vi "Create Case Structure (Boolean).vi"(0 "Diagram in":refnum<vi>, 2 "location (0, 0)":T1, 5 "Selector":refnum<vi>, 7 "Inputs":refnum<vi>[](array[refnum]), 11 "error in (no error)":errorcluster) -> (4 "Selected Diagram":refnum<vi>, 6 "Selector":refnum<vi>, 8 "Inputs":refnum<vi>[](array[refnum]), 15 "error out":errorcluster)   [LabVIEW 2015, in "Scripting.lvlib"]
doc: "Creates a Case Structure at <B>location</B> on <B>Diagram in</B> with True and False cases, in that order."
uses:
  Scripting.lvlib
  <vilib>/Utility/miscctls.llb/LVPointTypeDef.ctl
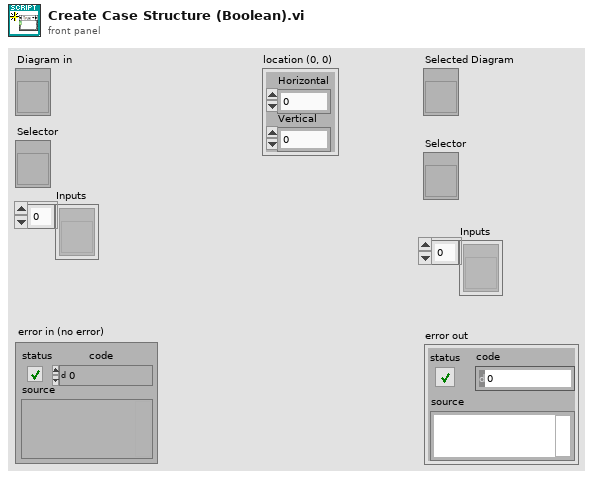
[diagram p1: front panel]
types:
  T1 = typedef "LVPointTypeDef.ctl" = cluster{"Horizontal":i16, "Vertical":i16}
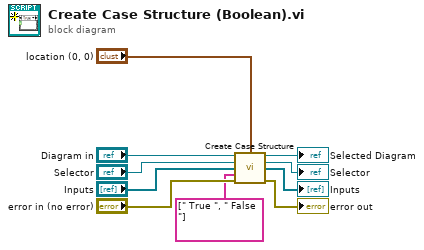
[diagram p0: block diagram]
diagram:
  n1 = call "Create Case Structure.vi"("Diagram in"="Diagram in", "location (0, 0)"="location (0, 0)", "Selector"="Selector", "Inputs"="Inputs", "Frames"=string[] [" True ", " False "], "error in (no error)"="error in (no error)") -> ("Selected Diagram"=→"Selected Diagram":refnum<vi>, "Selector"=→"Selector":refnum<vi>, "Inputs"=→"Inputs":refnum<vi>[], "error out"=→"error out":errorcluster)  [unwired: 6 in]
